vi "Write Path.vi"(8 "error in (no error)":errorcluster, 10 "Path":path, 11 "Text File in":refnum<class "Text File.lvclass">) -> (0 "error out":errorcluster, 3 "Text File out":refnum<class "Text File.lvclass">)   [LabVIEW 2020, in "Text File.lvlib" / "Text File.lvclass"]
uses:
  Text File.lvclass
  Text File.lvclass/Text File.ctl
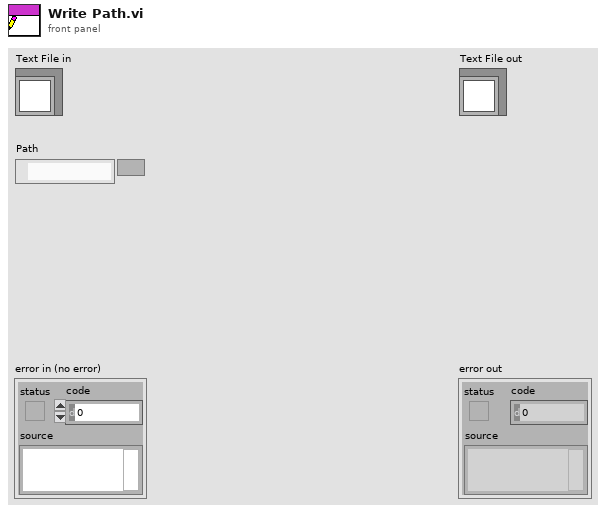
[diagram p1: front panel]
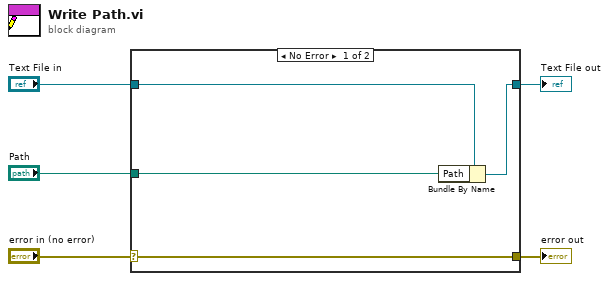
[diagram p0: block diagram]
diagram:
  n1 = case shown="No Error" "error in (no error)" {
    selector: "error in (no error)" -> [w9 w10]
    tunnel: [w9 w10] -> w4
    tunnel: [w7 w11] -> w2
    tunnel: "Text File in" -> [w8 w11]
    tunnel: "Path" -> [w6 _]
    frame No Error {
      n2 = Bundle By Name(cluster=w8, "Path"=w6) -> (w7:refnum<class "Text File.lvclass">)
    }
    frame Error {
    }
  }
  "error out" <- w4
  "Text File out" <- w2
